vi "ZeroOutputsTest.vi"() -> ()   [LabVIEW 2012]
uses:
  <vilib>/DAQmx/write.llb/DAQmx Write (Analog 1D DBL NChan 1Samp).vi
  <vilib>/DAQmx/create/channels.llb/DAQmx Create Channel (AO-Voltage-Basic).vi
  <vilib>/DAQmx/miscellaneous.llb/DAQmx Fill In Error Info.vi
  <resource>/objmgr/daqmx.rc
panel:
  out "SampTimingType":i32(ring)=10388 items=["Sample Clock"=10388, "Burst Handshake"=12548, "Handshake"=10389, "Implicit"=10451, "On Demand"=10390, "Change Detection"=12504, "Pipelined Sample Clock"=14668]
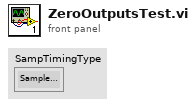
[diagram p1: front panel]
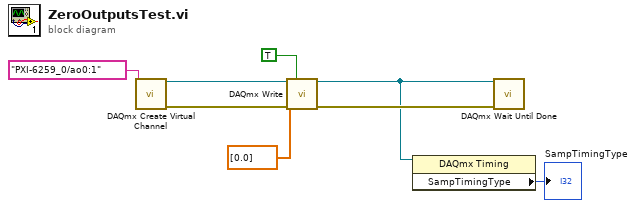
[diagram p0: block diagram]
diagram:
  n1 = call-poly <vilib>:"DAQmx Create Virtual Channel.vi"("physical channels"=tag "PXI-6259_0/ao0:1") -> ("task out"=w4:refnum<k21>, "error out"=w5:errorcluster)  [unwired: 13 in]
  n2 = call-poly <vilib>:"DAQmx Write.vi"("task/channels in"=w4, "auto start"=TRUE, "data"=dbl[] [0.0], "error in"=w5) -> ("task out"=w2:refnum<k21>, "error out"=w3:errorcluster)  [unwired: 9 in, 1 out]
  n3 = property class="DAQmx Timing"(reference=w2) -> ("SampTimingType"=→"SampTimingType":i32)  [unwired: 1 in, 2 out]
  n4 = call <vilib>:"DAQmx Wait Until Done.vi"("task/channels in"=w2, "error in"=w3) -> ()  [unwired: 12 in, 2 out]
